vi "WiiMote Read Accelerometer and Buttons.vi"(3 "error in":errorcluster, 4 "read raw values":bool, 5 "Wiimote":refnum<k24>) -> (0 "error out":errorcluster, 1 "Wiimote State":T1, 2 "reference out":refnum<k24>)   [LabVIEW 2013]
doc: "Get accel / button state from wiimote \nSam Shearman"
uses:
  WiiMote State.ctl
  D:/Users/jjensen/Documents/Lab Book/embeddedLab/exercises/LabVIEW/WiiMote/Dependencies/WiimoteLib.dll
  Dependencies/WiimoteLib.dll
panel:
  # "Establish a Bluetooth link with your Wiimote prior to executing this VI.\n\nRequires the Wiimote Managed Library WiimoteLib Ver 1.7\navailable from http://www.codeplex.com/WiimoteLib\nSam Shearman"
  # "Accelerometers"
  # "Buttons"
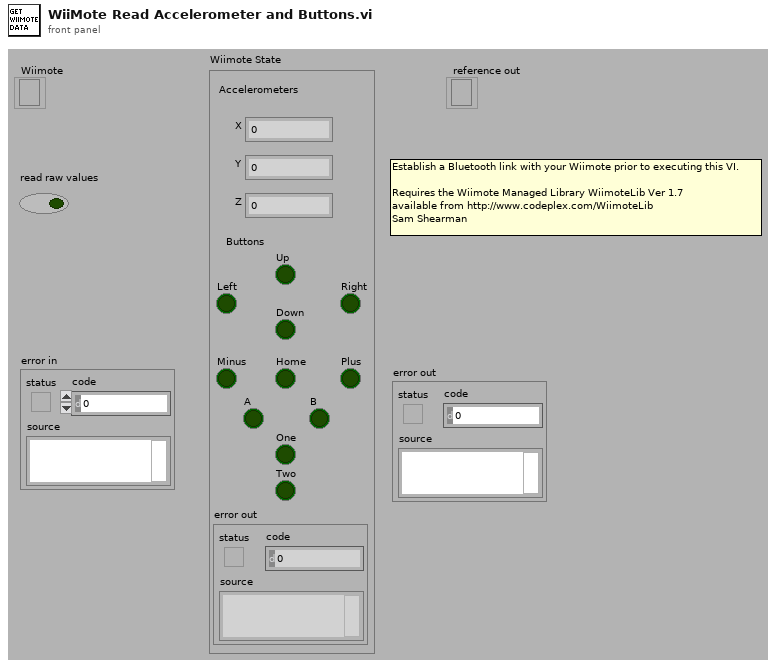
[diagram p1: front panel]
types:
  T1 = typedef "WiiMote State.ctl" = cluster{"X":sgl, "Y":sgl, "Z":sgl, "A":bool, "B":bool, "Down":bool, "Home":bool, "Left":bool, "Minus":bool, "One":bool, "Plus":bool, "Right":bool, "Two":bool, "Up":bool, "error out":errorcluster}
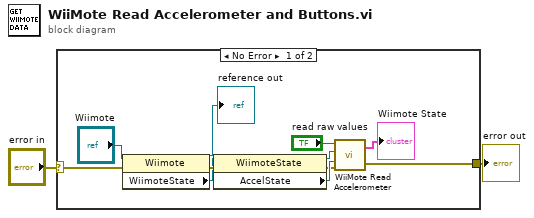
[diagram p0: block diagram]
diagram:
  n1 = case shown="No Error" "error in" {
    selector: "error in" -> [w10 w14]
    tunnel: [w5 w14] -> w2
    frame No Error {
      n2 = property class="Wiimote"(reference="Wiimote", error in=w10) -> (reference out=→"reference out":refnum<k24>, error out=w13:errorcluster, "WiimoteState"=w9:refnum<k24>)
      n3 = property class="WiimoteState"(reference=w9, error in=w13) -> (reference out=w7:refnum<k24>, error out=w4:errorcluster, "AccelState"=w8:refnum<k24>)
      n4 = call "WiiMote Read Accelerometer.vi"("error in"=w4, "AccelState"=w8, "WiimoteState"=w7, "read raw values"="read raw values") -> ("error out"=w5:errorcluster, "Wiimote State"=→"Wiimote State":T1)
    }
    frame Error {
    }
  }
  "error out" <- w2
